vi "报告打印.vi"(9 "输出簇":T1, 11 "打印?":bool) -> ()   [LabVIEW 2010]
uses:
  <vilib>/Utility/NIReport.llb/NI_report.lvclass
  <vilib>/Utility/NIReport.llb/Append Report Text (str wrap).vi
  全局量/试验配置信息.vi
  <vilib>/addons/_office/word.llb/Word Easy Table (str).vi
  <vilib>/addons/_office/NI_ReportGenerationToolkit.lvlib
panel:
  in  "序号":i32
  out "XY图":cluster{"Y":dbl[], "Y":dbl[]}[](graph)
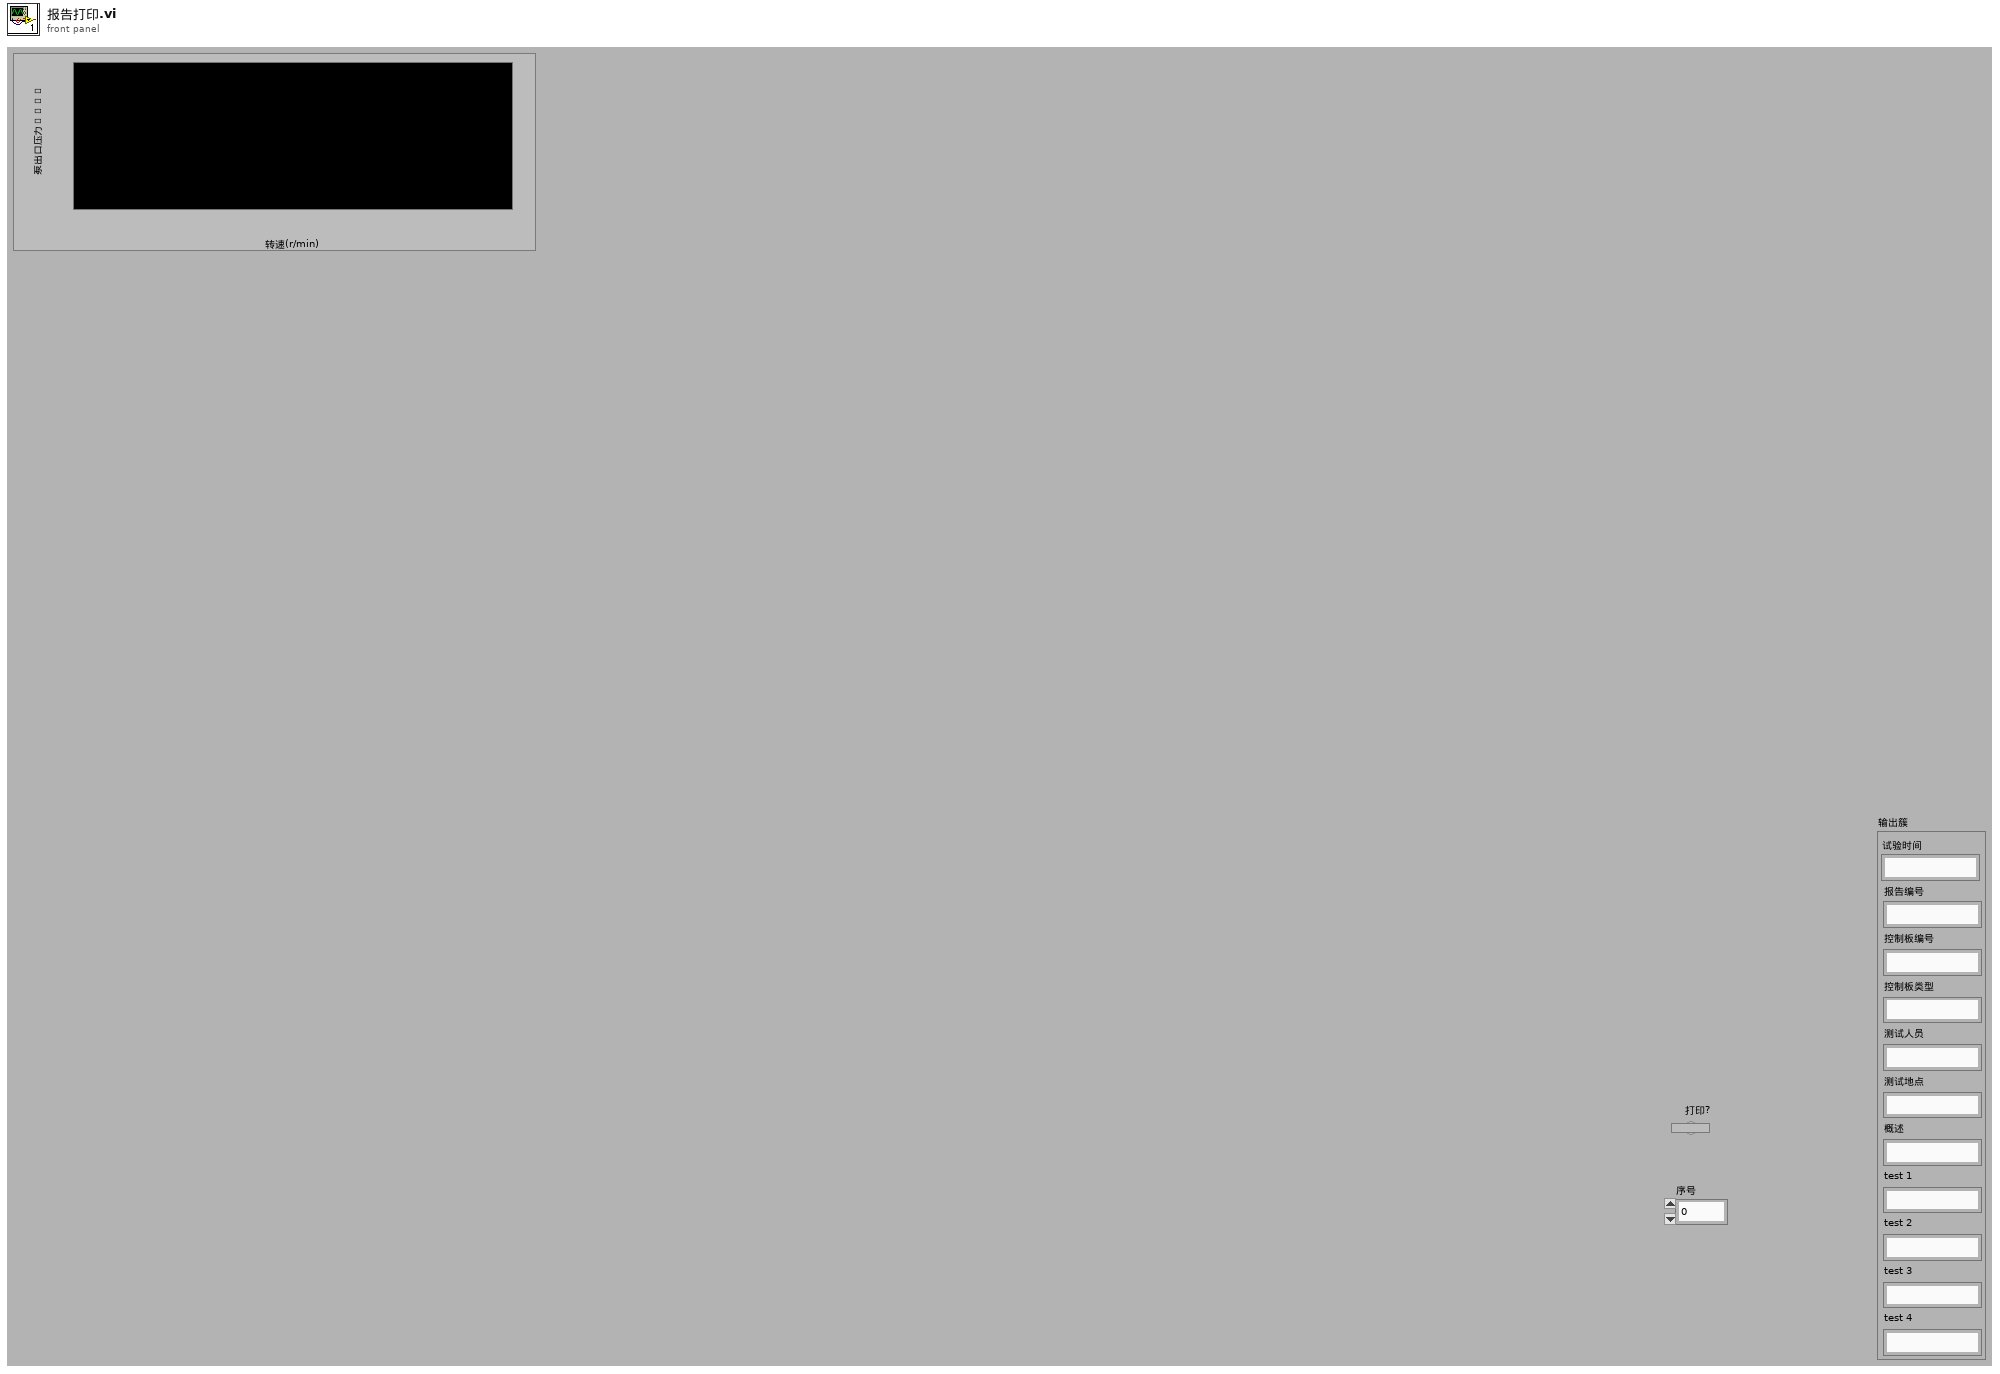
[diagram p1: front panel]
types:
  T1 = cluster{"试验时间":string, "报告编号":string, "控制板编号":string, "控制板类型":string, "测试人员":string, "测试地点":string, "概述":string, "test 1":string, "test 2":string, "test 3":string, "test 4":string}
  T2 = cluster{"position (Excel)":cluster{"row":i32, "column":i32}, "name (Excel)":string, "bookmark (Word)":string}
  T3 = enum16{"maximized", "minimized", "normal", "no change"}
  T4 = enum16{"Standard Report", "HTML", "Word", "Excel"}
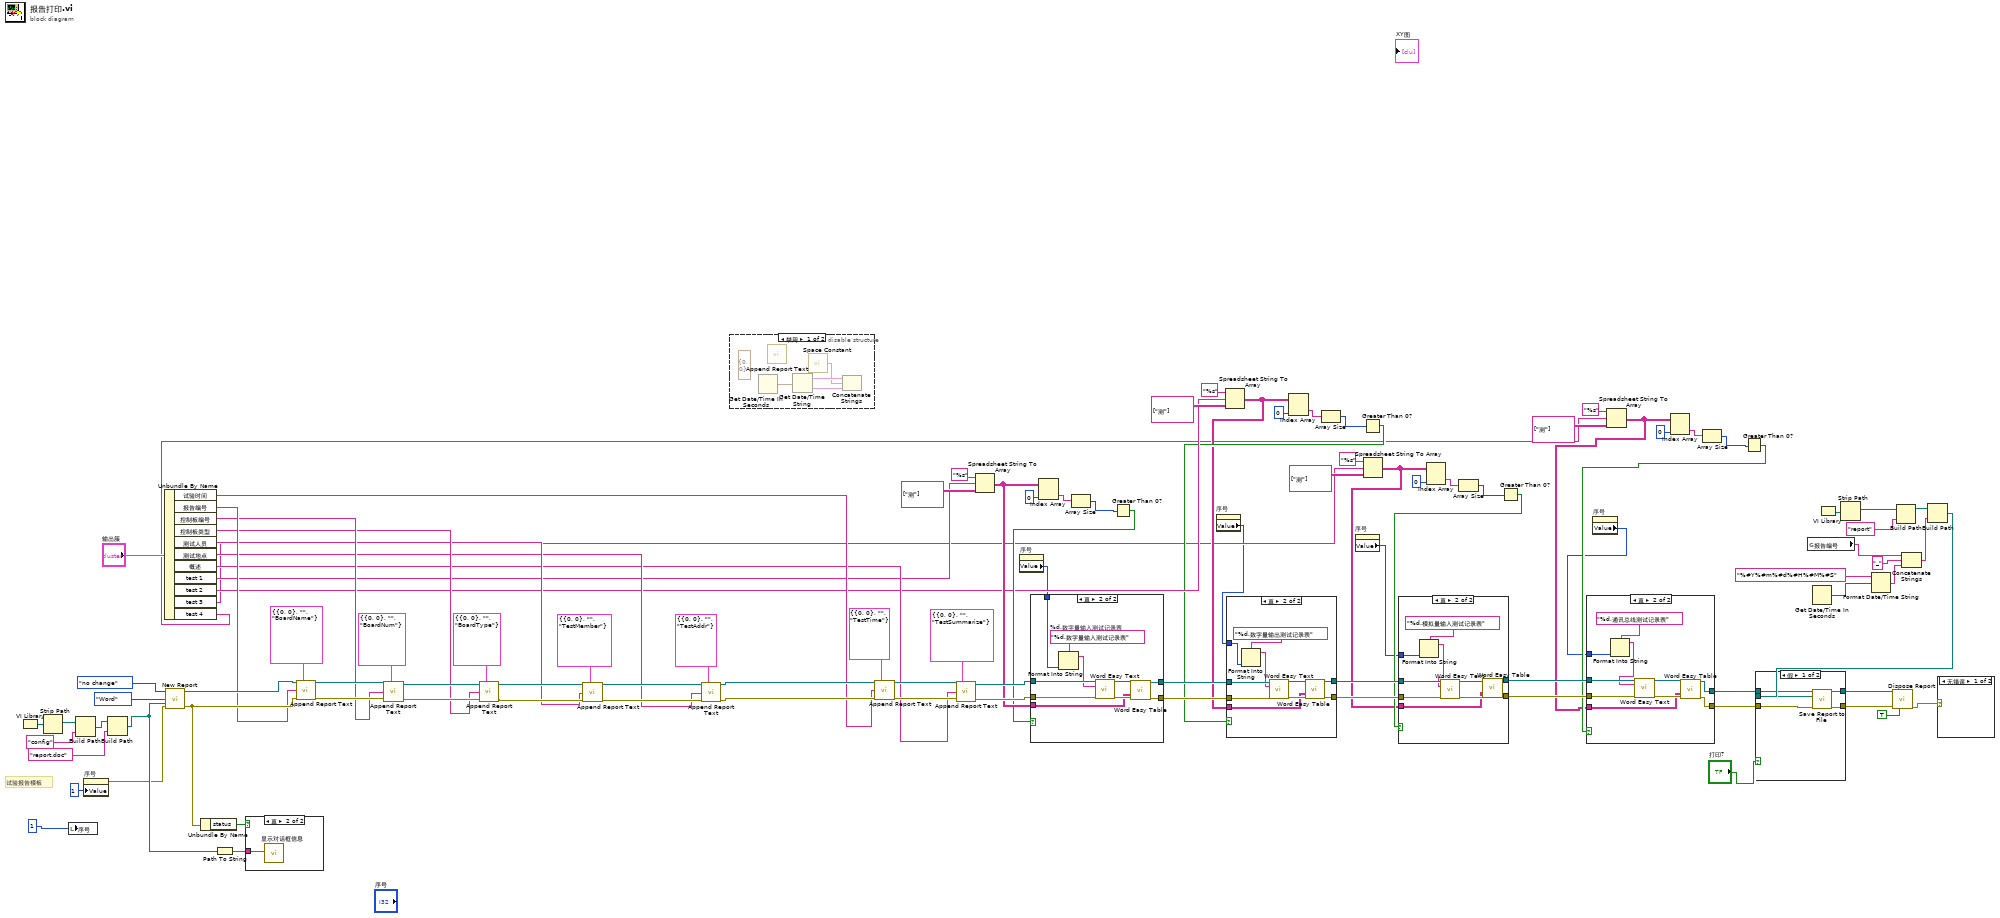
[diagram p0: block diagram]
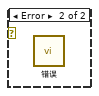
[diagram p6: hidden frame]
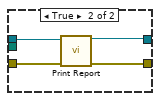
[diagram p7: hidden frame]
diagram:
  # "试验报告模板"
  n1 = VI Library() -> (path=w98:path)
  n2 = Strip Path(path=w98) -> (stripped path=w95:path)  [unwired: 1 out]
  n3 = local write "序号"(1) -> ()
  n4 = Build Path(base path=w95, name or relative path="config") -> (appended path=w97:path)
  n5 = property on="序号" class="DigNum (严格)"("Value"=1 ("序号")) -> (error out=w50:errorcluster)  [unwired: 2 in, 1 out]
  n6 = Build Path(base path=w97, name or relative path="report.doc") -> (appended path=w101:path)
  n7 = Unbundle By Name("输出簇") -> ("试验时间"=w40:string, "报告编号"=w45:string, "控制板编号"=w44:string, "控制板类型"=w43:string, "测试人员"=w42:string, "测试地点"=w41:string, "概述"=w39:string, "test 1"=w36:string, "test 2"=w26:string, "test 3"=w19:string, "test 4"=w12:string)
  n8 = call <vilib>:"New Report.vi"("window state (normal)"=T3."no change", "report type"=T4."Word", "template (empty)"=w101, "error in (no error)"=w50) -> ("report out"=w92:refnum<class "NI_report.lvclass">, "error out"=w91:errorcluster)  [unwired: 10 in]
  n9 = Unbundle By Name(w91) -> ("status"=w103:bool)
  n10 = Path To String(path=w101) -> (string=w102:string)
  n11 = case shown="真" w103 {
    tunnel: w102 -> [_ w105]
    frame False {
    }
    frame True {
      n12 = call "显示对话框信息"("Message"=w105) -> ()  [unwired: 9 in, 2 out]
    }
  }
  n13 = call-poly <vilib>:"Append Report Text.vi"("report in"=w92, "MS Office parameters"=T2 {"position (Excel)"={"row"=0, "column"=0}, "name (Excel)"="", "bookmark (Word)"="BoardName"}, "text"=w45, "error in (no error)"=w91) -> ("report out"=w77:refnum<class "NI_report.lvclass">, "error out"=w76:errorcluster)  [unwired: 8 in, 2 out]
  n14 = call-poly <vilib>:"Append Report Text.vi"("report in"=w77, "MS Office parameters"=T2 {"position (Excel)"={"row"=0, "column"=0}, "name (Excel)"="", "bookmark (Word)"="BoardNum"}, "text"=w44, "error in (no error)"=w76) -> ("report out"=w87:refnum<class "NI_report.lvclass">, "error out"=w86:errorcluster)  [unwired: 8 in, 2 out]
  n15 = call-poly <vilib>:"Append Report Text.vi"("report in"=w87, "MS Office parameters"=T2 {"position (Excel)"={"row"=0, "column"=0}, "name (Excel)"="", "bookmark (Word)"="BoardType"}, "text"=w43, "error in (no error)"=w86) -> ("report out"=w84:refnum<class "NI_report.lvclass">, "error out"=w83:errorcluster)  [unwired: 8 in, 2 out]
  n16 = call-poly <vilib>:"Append Report Text.vi"("report in"=w84, "MS Office parameters"=T2 {"position (Excel)"={"row"=0, "column"=0}, "name (Excel)"="", "bookmark (Word)"="TestMember"}, "text"=w42, "error in (no error)"=w83) -> ("report out"=w81:refnum<class "NI_report.lvclass">, "error out"=w80:errorcluster)  [unwired: 8 in, 2 out]
  n17 = call-poly <vilib>:"Append Report Text.vi"("report in"=w81, "MS Office parameters"=T2 {"position (Excel)"={"row"=0, "column"=0}, "name (Excel)"="", "bookmark (Word)"="TestAddr"}, "text"=w41, "error in (no error)"=w80) -> ("report out"=w79:refnum<class "NI_report.lvclass">, "error out"=w78:errorcluster)  [unwired: 8 in, 2 out]
  n18 = disable-structure shown="禁用" {
    frame Disabled {
      (unwired) cluster{"row":i32, "column":i32} {"row"=0, "column"=0} ("position (excel)")
      n19 = Get Date/Time In Seconds() -> (seconds since 1Jan1904=w109:timestamp)
      n20 = call-poly <vilib>:"Append Report Text.vi"() -> ()  [unwired: 12 in, 4 out]
      n21 = Get Date/Time String(seconds (now)=w109) -> (date string=w108:string, time string=w107:string)  [unwired: 2 in]
      n22 = call <vilib>:"Space Constant.vi"() -> ("String"=w106:string)
      n23 = Concatenate Strings(w108, w106, w107) -> ()  [unwired: 1 out]
    }
    frame Enabled {
    }
  }
  n24 = call-poly <vilib>:"Append Report Text.vi"("report in"=w79, "MS Office parameters"=T2 {"position (Excel)"={"row"=0, "column"=0}, "name (Excel)"="", "bookmark (Word)"="TestTime"}, "text"=w40, "error in (no error)"=w78) -> ("report out"=w55:refnum<class "NI_report.lvclass">, "error out"=w54:errorcluster)  [unwired: 8 in, 2 out]
  n25 = call-poly <vilib>:"Append Report Text.vi"("report in"=w55, "MS Office parameters"=T2 {"position (Excel)"={"row"=0, "column"=0}, "name (Excel)"="", "bookmark (Word)"="TestSummarize"}, "text"=w39, "error in (no error)"=w54) -> ("report out"=w53:refnum<class "NI_report.lvclass">, "error out"=w52:errorcluster)  [unwired: 8 in, 2 out]
  n26 = Spreadsheet String To Array(format string="%s" ("格式字符串"), spreadsheet string=w36, array type (2D Dbl)=string[][] [["测"]] ("数组类型(2D String)")) -> (array=w35:string[][])  [unwired: 1 in]
  n27 = property on="序号" class="DigNum (严格)"() -> ("Value"=w8:i32)  [unwired: 2 in, 2 out]
  n28 = Index Array(array=w35, index (col)=0 ("禁用的索引 (列)")) -> (element=w33:string[])  [unwired: 1 in]
  n29 = Array Size(array=w33) -> (size(s)=w32:i32)
  n30 = Greater Than 0?(x=w32) -> (x > 0?=w31:bool)
  n31 = case shown="真" w31 {
    tunnel: [w111 w120] -> w62
    tunnel: [w110 w119] -> w60
    tunnel: w53 -> [w111 w117]
    tunnel: w52 -> [w110 w116]
    tunnel: w35 -> [_ w113]
    tunnel: w8 -> [_ w112]
    frame False {
    }
    frame True {
      w115 = "%d.数字量输入测试记录表"  # %d.数字量输入测试记录表
      n32 = Format Into String(format string=w115, w112) -> (resulting string=w114:string)  [unwired: 2 in, 1 out]
      n33 = call <vilib>:"Word Easy Text.vi"("report in"=w117, "text"=w114, "error in (no error)"=w116) -> ("report out"=w121:refnum<class "NI_report.lvclass">, "error out"=w118:errorcluster)  [unwired: 10 in, 1 out]
      n34 = call-poly <vilib>:"Word Easy Table.vi"("report in"=w121, "data"=w113, "error in (no error)"=w118) -> ("report out"=w120:refnum<class "NI_report.lvclass">, "error out"=w119:errorcluster)  [unwired: 10 in, 1 out]
    }
  }
  n35 = property on="序号" class="DigNum (严格)"() -> ("Value"=w7:i32)  [unwired: 2 in, 2 out]
  n36 = Spreadsheet String To Array(format string="%s" ("格式字符串"), spreadsheet string=w26, array type (2D Dbl)=string[][] [["测"]] ("数组类型(2D String)")) -> (array=w24:string[][])  [unwired: 1 in]
  n37 = Index Array(array=w24, index (col)=0 ("禁用的索引 (列)")) -> (element=w27:string[])  [unwired: 1 in]
  n38 = Array Size(array=w27) -> (size(s)=w6:i32)
  n39 = property on="序号" class="DigNum (严格)"() -> ("Value"=w5:i32)  [unwired: 2 in, 2 out]
  n40 = Greater Than 0?(x=w6) -> (x > 0?=w25:bool)
  n41 = case shown="真" w25 {
    tunnel: w62 -> [w123 w133]
    tunnel: [w123 w131] -> w61
    tunnel: w60 -> [w122 w130]
    tunnel: [w122 w128] -> w59
    tunnel: w7 -> [_ w125]
    tunnel: w24 -> [_ w124]
    frame False {
    }
    frame True {
      n42 = Format Into String(format string="%d.数字量输出测试记录表", w125) -> (resulting string=w126:string)  [unwired: 2 in, 1 out]
      n43 = call <vilib>:"Word Easy Text.vi"("report in"=w133, "text"=w126, "error in (no error)"=w130) -> ("report out"=w132:refnum<class "NI_report.lvclass">, "error out"=w129:errorcluster)  [unwired: 10 in, 1 out]
      n44 = call-poly <vilib>:"Word Easy Table.vi"("report in"=w132, "data"=w124, "error in (no error)"=w129) -> ("report out"=w131:refnum<class "NI_report.lvclass">, "error out"=w128:errorcluster)  [unwired: 10 in, 1 out]
    }
  }
  n45 = Spreadsheet String To Array(format string="%s" ("格式字符串"), spreadsheet string=w19, array type (2D Dbl)=string[][] [["测"]] ("数组类型(2D String)")) -> (array=w17:string[][])  [unwired: 1 in]
  n46 = Index Array(array=w17, index (col)=0 ("禁用的索引 (列)")) -> (element=w20:string[])  [unwired: 1 in]
  n47 = Array Size(array=w20) -> (size(s)=w4:i32)
  n48 = Greater Than 0?(x=w4) -> (x > 0?=w18:bool)
  n49 = case shown="真" w18 {
    tunnel: w61 -> [w135 w145]
    tunnel: w59 -> [w134 w143]
    tunnel: [w135 w141] -> w58
    tunnel: [w134 w140] -> w57
    tunnel: w5 -> [_ w137]
    tunnel: w17 -> [_ w136]
    frame False {
    }
    frame True {
      n50 = Format Into String(format string="%d.模拟量输入测试记录表", w137) -> (resulting string=w138:string)  [unwired: 2 in, 1 out]
      n51 = call <vilib>:"Word Easy Text.vi"("report in"=w145, "text"=w138, "error in (no error)"=w143) -> ("report out"=w144:refnum<class "NI_report.lvclass">, "error out"=w142:errorcluster)  [unwired: 10 in, 1 out]
      n52 = call-poly <vilib>:"Word Easy Table.vi"("report in"=w144, "data"=w136, "error in (no error)"=w142) -> ("report out"=w141:refnum<class "NI_report.lvclass">, "error out"=w140:errorcluster)  [unwired: 10 in, 1 out]
    }
  }
  n53 = property on="序号" class="DigNum (严格)"() -> ("Value"=w3:i32)  [unwired: 2 in, 2 out]
  n54 = Spreadsheet String To Array(format string="%s" ("格式字符串"), spreadsheet string=w12, array type (2D Dbl)=string[][] [["测"]] ("数组类型(2D String)")) -> (array=w10:string[][])  [unwired: 1 in]
  n55 = Index Array(array=w10, index (col)=0 ("禁用的索引 (列)")) -> (element=w13:string[])  [unwired: 1 in]
  n56 = Array Size(array=w13) -> (size(s)=w2:i32)
  n57 = Greater Than 0?(x=w2) -> (x > 0?=w11:bool)
  n58 = case shown="真" w11 {
    tunnel: [w147 w157] -> w64
    tunnel: [w146 w156] -> w63
    tunnel: w58 -> [w147 w155]
    tunnel: w57 -> [w146 w154]
    tunnel: w3 -> [_ w149]
    tunnel: w10 -> [_ w148]
    frame False {
    }
    frame True {
      n59 = Format Into String(format string="%d.通讯总线测试记录表", w149) -> (resulting string=w150:string)  [unwired: 2 in, 1 out]
      n60 = call <vilib>:"Word Easy Text.vi"("report in"=w155, "text"=w150, "error in (no error)"=w154) -> ("report out"=w153:refnum<class "NI_report.lvclass">, "error out"=w152:errorcluster)  [unwired: 10 in, 1 out]
      n61 = call-poly <vilib>:"Word Easy Table.vi"("report in"=w153, "data"=w148, "error in (no error)"=w152) -> ("report out"=w157:refnum<class "NI_report.lvclass">, "error out"=w156:errorcluster)  [unwired: 10 in, 1 out]
    }
  }
  n62 = global read "试验配置信息.vi" "报告编号"() -> (w48:string)
  n63 = Get Date/Time In Seconds() -> (seconds since 1Jan1904=w70:timestamp)
  n64 = VI Library() -> (path=w71:path)
  n65 = Strip Path(path=w71) -> (stripped path=w74:path)  [unwired: 1 out]
  n66 = Format Date/Time String(time format string (%c)="%#Y%#m%#d%#H%#M%#S" ("时间格式字符串(%c)"), seconds (now)=w70) -> (date/time string=w49:string)  [unwired: 1 in]
  n67 = Build Path(base path=w74, name or relative path="report") -> (appended path=w72:path)
  n68 = Concatenate Strings(w48, "_", w49) -> (w46:string)
  n69 = Build Path(base path=w72, name or relative path=w46) -> (appended path=w66:path)
  n70 = case shown="假" "打印?" {
    tunnel: w64 -> [w162 w166]
    tunnel: w63 -> [w161 w165]
    tunnel: [w160 w164] -> w68
    tunnel: [w159 w163] -> w67
    tunnel: w66 -> [w158 _]
    frame False {
      n71 = call-dynamic "Save Report to File.vi"("report in"=w162, "report file path"=w158, "error in (no error)"=w161) -> ("report out"=w160:refnum<class "NI_report.lvclass">, "error out"=w159:errorcluster)  [unwired: 11 in]
    }
    frame True {
      n72 = call-dynamic "Print Report.vi"("report in"=w166, "error in (no error)"=w165) -> ("report out"=w164:refnum<class "NI_report.lvclass">, "error out"=w163:errorcluster)  [unwired: 12 in]
    }
  }
  n73 = call-dynamic "Dispose Report.vi"("report in"=w68, "error in (no error)"=w67, "close report? (T)"=TRUE) -> ("error out"=w65:errorcluster)  [unwired: 12 in]
  n74 = case shown="无错误" w65 {
    frame No Error {
    }
    frame Error {
      n75 = call "错误"() -> ()  [unwired: 10 in, 2 out]
    }
  }
